vi "SLSC Session Property Node.vi"   [LabVIEW 2020]
doc: "A Property Node with the SLSC Session class preselected. Property nodes may be used to access properties that are defined by the SLSC driver, but cannot be used to access properties that are defined by SLSC devices."
uses:
  <resource>/objmgr/slsc.rc
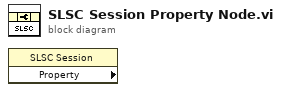
[diagram p0: block diagram]
diagram:
  n1 = property class="SLSC Session" props=[]() -> ()  [unwired: 2 in, 3 out]
